vi "例程37-基本平均直流-均方根VI的使用.vi"() -> ()   [LabVIEW 2016]
uses:
  <vilib>/measure/madcrms.llb/Basic Averaged DC-RMS for 1 Chan.vi
  <vilib>/measure/NI_MABase.lvlib
  <vilib>/measure/NI_MAPro.lvlib
panel:
  in  "停止":bool
  out "波形图":waveform(dbl)(graph)={"t0"=timestamp(186574.0 s since 1904-01-01), "dt"=0.001, "Y"=array[1000 elements]}
  out "RMS value":dbl=1.2247448700000008 caption="均方根值" format="%0.2p"
  out "DC value":dbl=0.9999999999999999 caption="直流值" format="%0.2p"
  in  "window":T1(ring)=enum."Hanning" caption="窗"
  in  "averaging type":enum16{"Linear", "Exponential"}(ring) caption="平均类型"
  in  "square wave duty cycle (%)":dbl=50.0 caption="方波占空比(%)" format="%0.2f"
  in  "offset":dbl=1.0 caption="偏移量" format="%0.2p"
  in  "signal type":T2(ring) caption="信号类型"
  in  "phase":dbl caption="相位" format="%.2p"
  in  "amplitude":dbl=1.0 caption="幅值" format="%0.2p"
  in  "frequency":dbl=10.0 caption="频率" format="%0.2p"
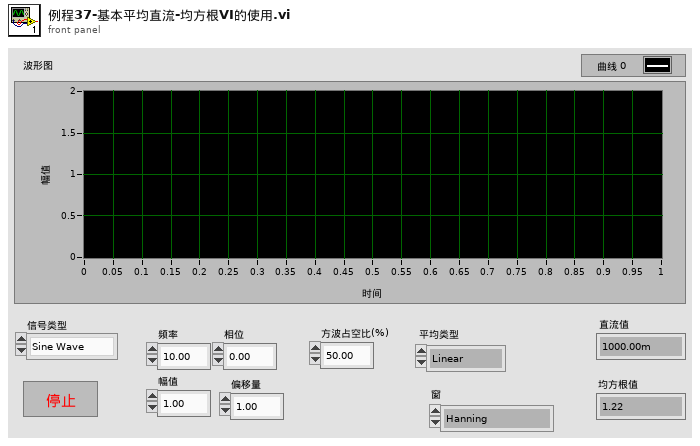
[diagram p1: front panel]
types:
  T1 = enum16{"Rectangular (none)", "Hanning", "Low side lobe"}
  T2 = enum16{"Sine Wave", "Triangle Wave", "Square Wave", "Sawtooth Wave"}
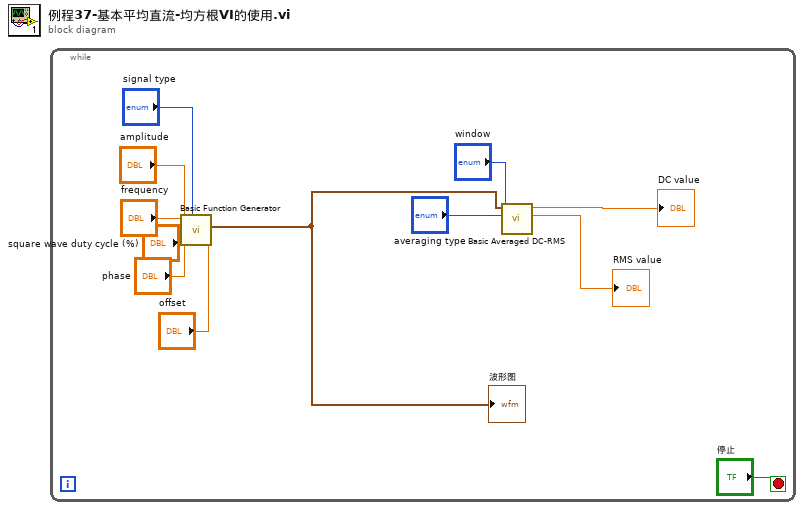
[diagram p0: block diagram]
diagram:
  n1 = while {
    stop <- "停止" stop-if-true
    n2 = call <vilib>:"Basic Function Generator.vi"("offset"="offset", "square wave duty cycle (%)"="square wave duty cycle (%)", "signal type"="signal type", "phase"="phase", "amplitude"="amplitude", "frequency"="frequency") -> ("signal out"=w2:waveform(dbl))  [unwired: 3 in, 2 out]
    "波形图" <- w2
    n3 = call-poly <vilib>:"Basic Averaged DC-RMS.vi"("window"="window", "averaging type"="averaging type", "signal in"=w2) -> ("RMS value"=→"RMS value":dbl, "DC value"=→"DC value":dbl)  [unwired: 5 in, 2 out]
  }
